vi "OP500Z8_Plus1OuCrash.vi"(2 "IsStepOK?":bool, 3 "in":T1) -> (0 "Out":T1=enum."CRASH")   [LabVIEW 2020]
uses:
  navZENPLUS.ctl
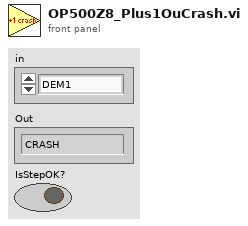
[diagram p1: front panel]
types:
  T1 = typedef "navZENPLUS.ctl" = enum8{"DEM1", "Init", "DEM2", "SCAN", "SECU", "OCVACIR", "Montage", "GoInsuPlus", "InsulationBplus", "GoInsuMoins", "InsulationBmoins", "GoDCIR", "DCIR", "Collage PAD", "Demontage", "CLOSE", "extinction", "CRASH"}
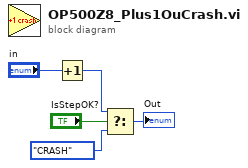
[diagram p0: block diagram]
diagram:
  n1 = Increment(x="in") -> (x+1=w4:T1)
  n2 = Select(t=w4, s="IsStepOK?", f=navZENPLUS."CRASH") -> (s? t:f=→"Out":T1)
